vi "stepper driver -- IMS.vi"(6 "Instrument Address":refnum<visa-resource-name>="ASRL2::INSTR", 7 "stepper driver action":T1, 10 "speed IN":dbl, 11 "number":dbl format="%#_13g") -> (1 "stepper motor state OUT":T2, 2 "speed":dbl, 3 "number out":dbl)   [LabVIEW 2018]
uses:
  stepper motor state.ctl
  stepper driver action.ctl
  internal stepper driver state -- IMS.ctl
  Q - not nan -- integer.vi
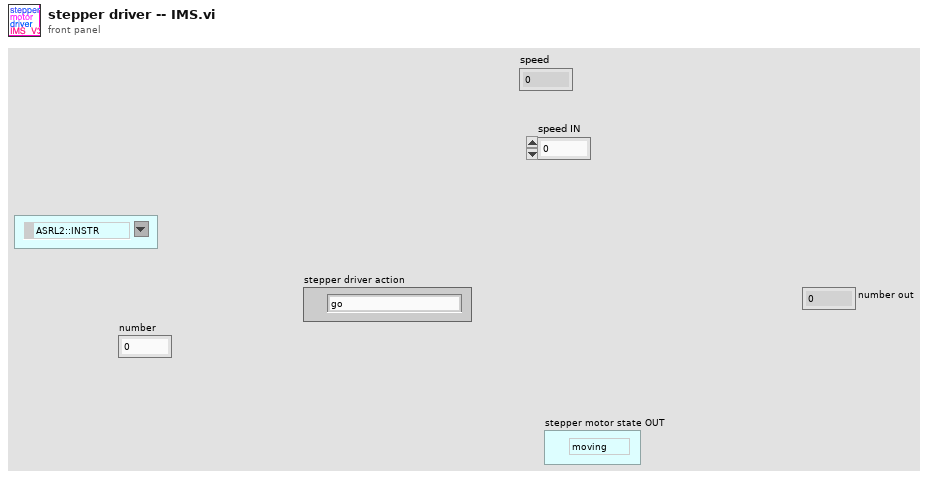
[diagram p1: front panel]
types:
  T1 = typedef "stepper driver action.ctl" = enum16{"go", "void", "stop", "check", "init", "sync", "set", "set speed", "--check status", "--check value"}
  T2 = typedef "stepper motor state.ctl" = enum16{"moving", "stopped"}
  T3 = typedef "internal stepper driver state -- IMS.ctl" = cluster{"VISA address":refnum<visa-resource-name>, "stepper motor state":T2, "Motor Address":u32, "speed":i32, "target position":dbl, "current position":dbl}
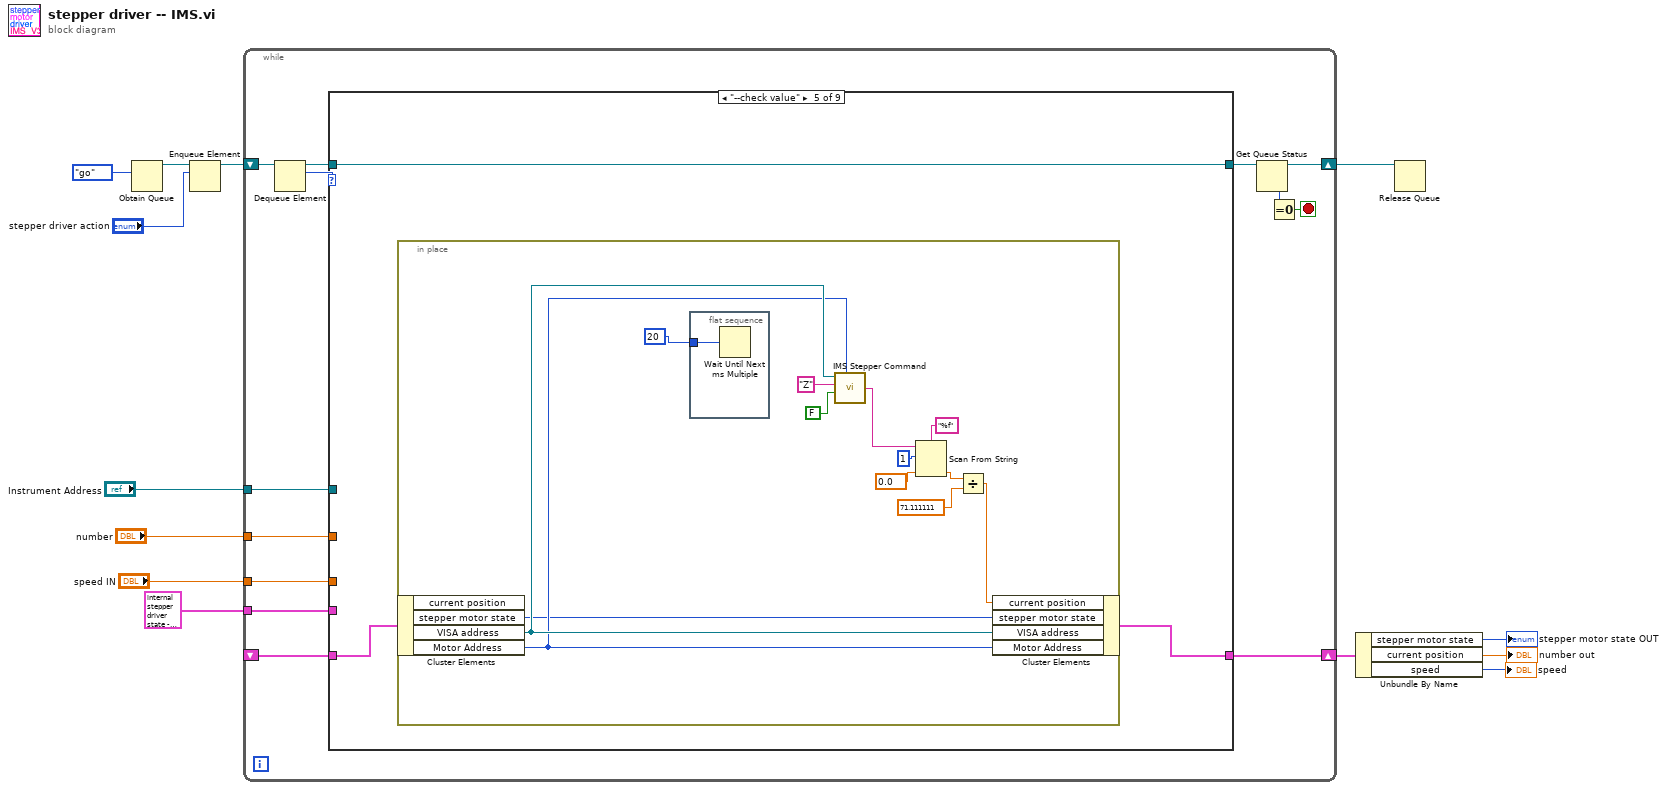
[diagram p0: block diagram]
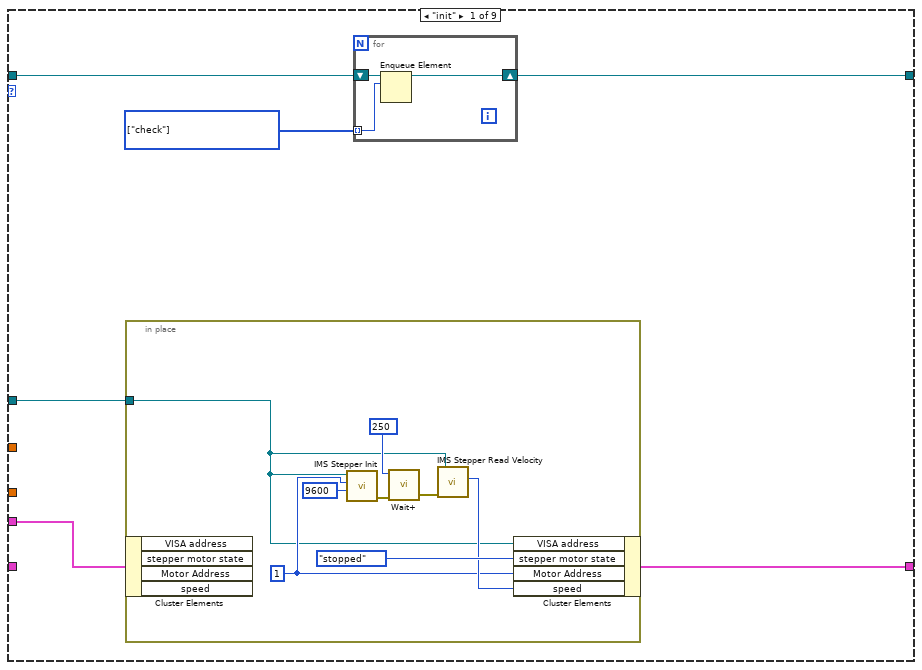
[diagram p2: hidden frame]
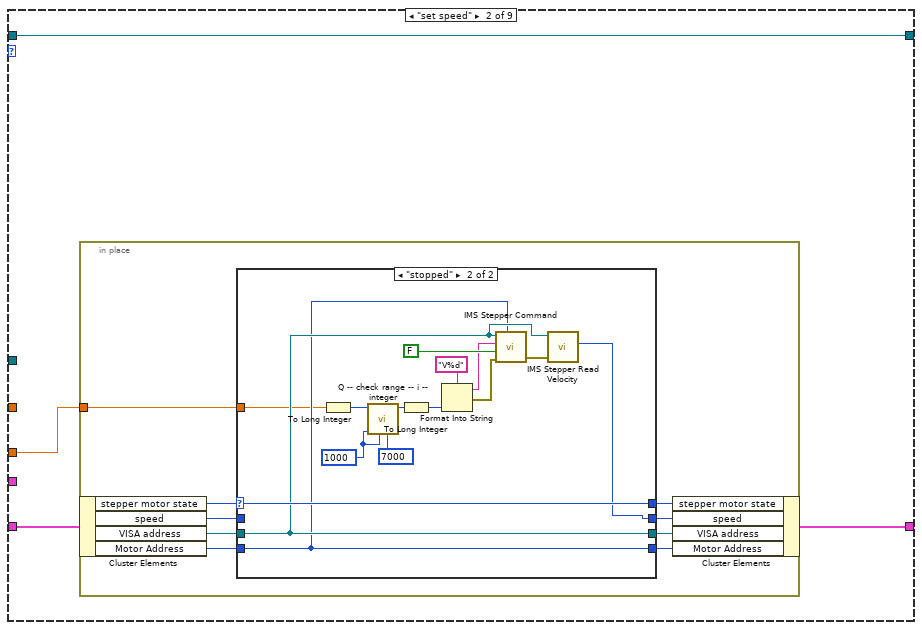
[diagram p3: hidden frame]
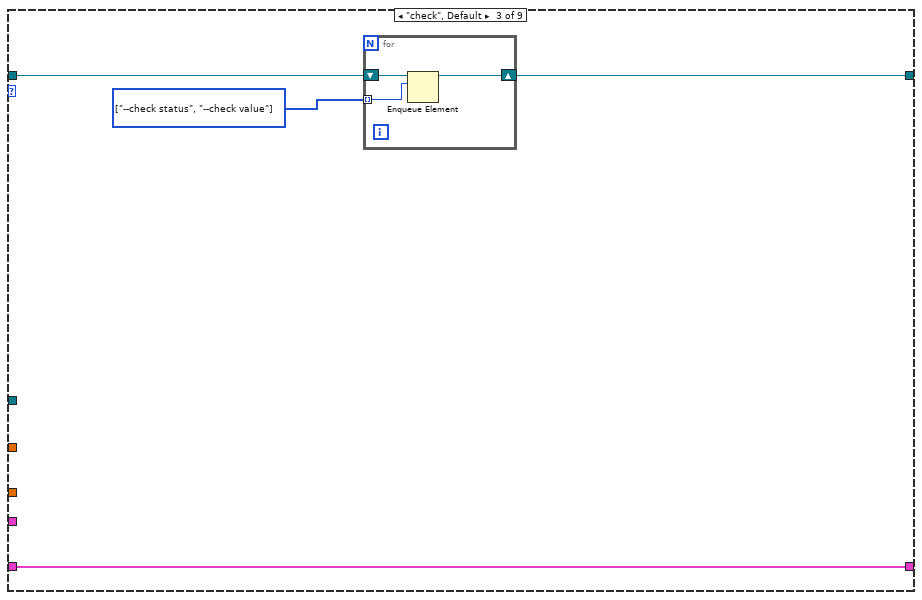
[diagram p5: hidden frame]
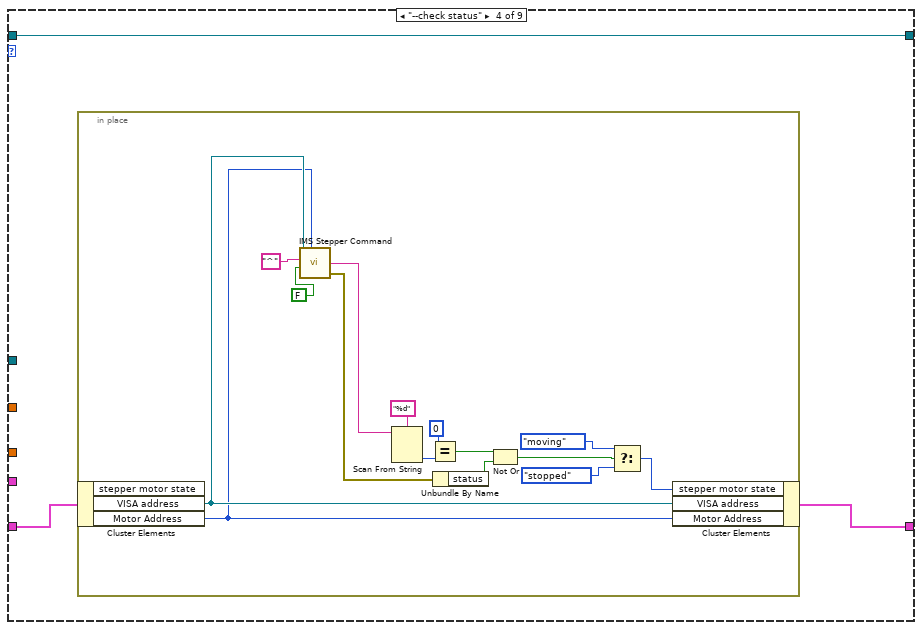
[diagram p6: hidden frame]
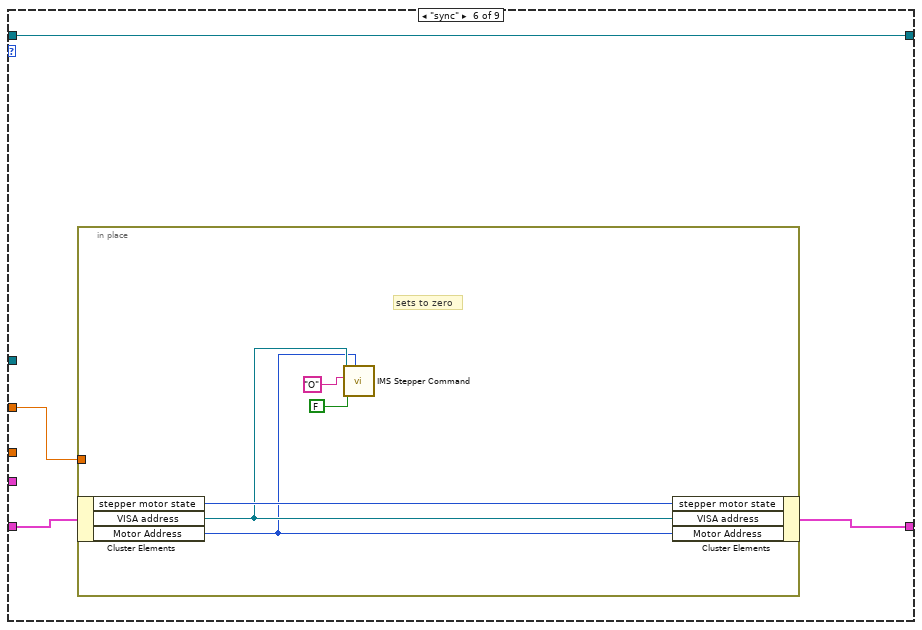
[diagram p7: hidden frame]
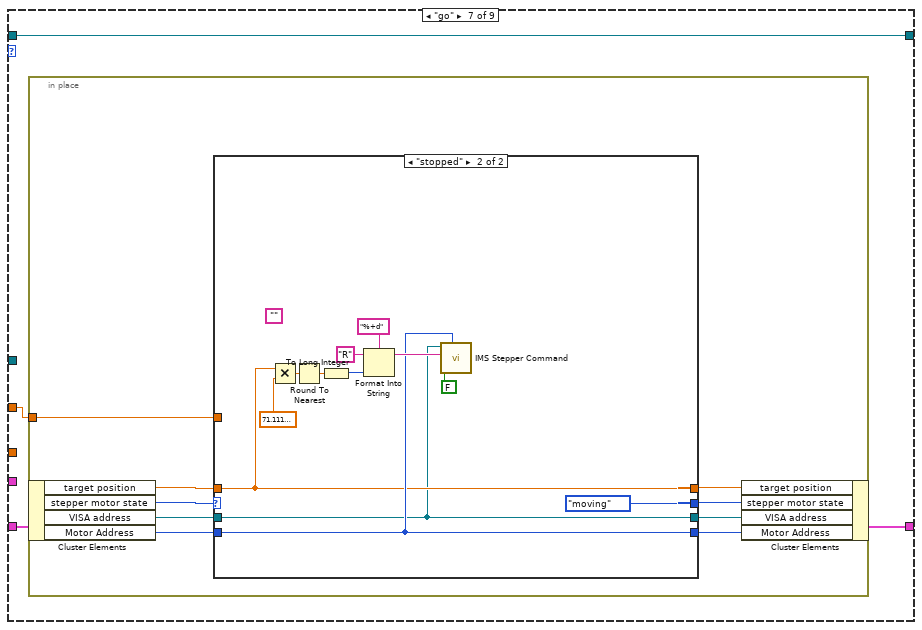
[diagram p8: hidden frame]
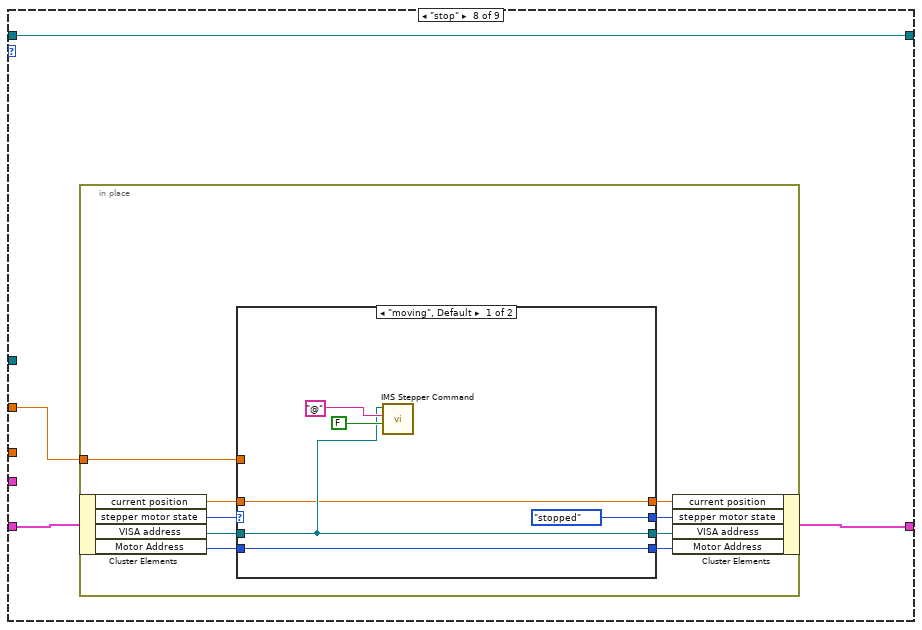
[diagram p10: hidden frame]
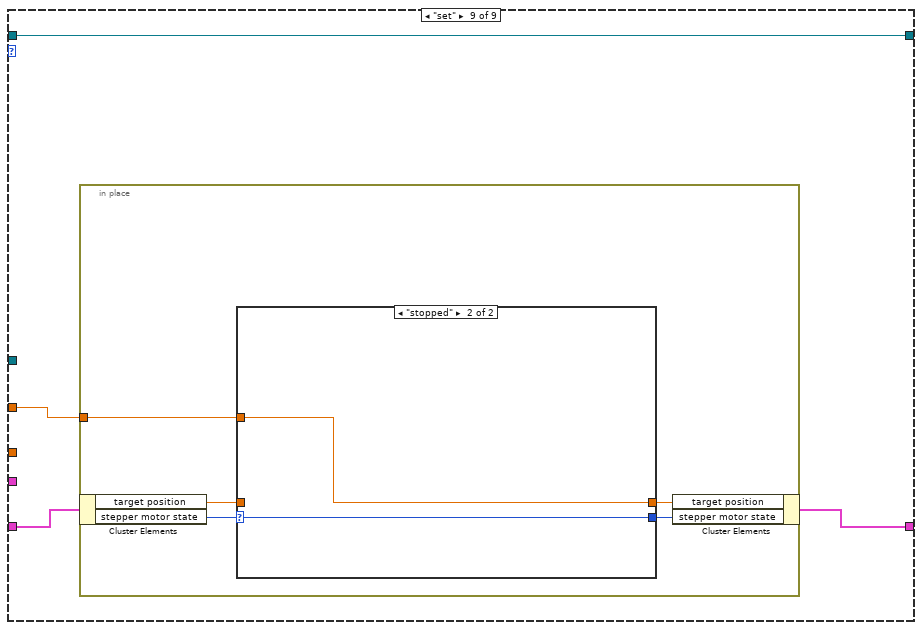
[diagram p12: hidden frame]
diagram:
  n1 = Obtain Queue(element data type=stepper_driver_action."go" ("stepper driver action")) -> (queue out=w8:refnum<queue>)  [unwired: 4 in, 2 out]
  n2 = Enqueue Element(queue=w8, element="stepper driver action") -> (queue out=w7:refnum<queue>)  [unwired: 2 in, 2 out]
  n3 = while {
    shift-right: [w26] -> w10
    shift-left: _ -> [w25]
    shift-right: [w18] -> w6
    shift-left: w7 -> [w22]
    tunnel: T3 {"VISA address"="GPIB0::25::INSTR", "stepper motor state"=enum."stopped", "Motor Address"=0, "speed"=0, "target position"=0.0, "current position"=0.0} ("internal stepper driver state IMS") -> [w24]
    tunnel: "number" -> [w23]
    tunnel: "Instrument Address" -> [w15]
    tunnel: "speed IN" -> [w14]
    stop <- w16 stop-if-true
    n4 = Dequeue Element(queue=w22) -> (queue out=w21:refnum<queue>, element=w20:T1)  [unwired: 2 in, 2 out]
    n5 = case shown="\"--check value\"" w20 {
      tunnel: [w31 w45 w79 w84 w102 w119 w128 w157 w180] -> w26
      tunnel: w25 -> [_ w46 w79 w85 w103 w120 w129 w158 w181]
      tunnel: [w29 w47 w77 w83 w101 w121 w130 w159 w182] -> w19
      tunnel: w21 -> [w30 w47 w78 w83 w101 w121 w130 w159 w182]
      tunnel: w24 -> [w32 _ _ _ _ _ _ _ _]
      tunnel: w23 -> [_ _ _ _ _ w118 w127 w156 w179]
      tunnel: w15 -> [w27 _ _ _ _ _ _ _ _]
      tunnel: w14 -> [_ w44 _ _ _ _ _ _ _]
      frame "init" {
        w28 = T1[] [enum."check"] items=["go", "void", "stop", "check", "init", "sync", "set", "set speed", "--check status", "--check value"] ("action list IN")
        n6 = in-place {
          in-place-border: w27 -> [w36]
          w37 = u32 1 ("Motor Address")
          n7 = in-place-cluster #1(w32) -> ()  [unwired: 4 out]
          n8 = call "IMS Stepper Init.vi"("Baud Rate"=u32 9600, "Motor Number"=w37, "Instrument Address"=w36) -> ("error out"=w42:errorcluster)  [unwired: 1 in, 1 out]
          n9 = call "Wait+.vi"("Error In"=w42, "milliseconds to wait"=u32 250) -> ("Error Out"=w41:errorcluster)  [unwired: 4 in, 1 out]
          n10 = call "IMS Stepper Read Velocity.vi"("error in (no error)"=w41, "Instrument Address"=w36) -> ("Velocity"=w38:i32)  [unwired: 3 in, 2 out]
          n11 = in-place-cluster #1("VISA address"=w36, "stepper motor state"=stepper_motor_state."stopped", "Motor Address"=w37, "speed"=w38) -> (w31:T3)
        }
        n12 = for {
          shift-right: [w34] -> w29
          shift-left: w30 -> [w35]
          tunnel: w28 -> [w33] mode=indexing
          n13 = Enqueue Element(queue=w35, element=w33) -> (queue out=w34:refnum<queue>)  [unwired: 2 in, 2 out]
        }
      }
      frame "set speed" {
        n14 = in-place {
          in-place-border: w44 -> [w56]
          n15 = in-place-cluster #2(w46) -> ("stepper motor state"=w52:T2, "speed"=w51:i32, "VISA address"=w54:refnum<visa-resource-name>, "Motor Address"=w53:u32)
          n16 = case shown="\"stopped\"" w52 {
            selector: w52 -> [w57 w73]
            tunnel: w56 -> [_ w62]
            tunnel: [w60 w64] -> w55
            tunnel: w54 -> [w59 w65]
            tunnel: w53 -> [w58 w63]
            tunnel: w51 -> [w60 _]
            tunnel: [w59 w65] -> w50
            tunnel: [w58 w63] -> w49
            tunnel: [w57 w73] -> w48
            frame "moving", Default {
            }
            frame "stopped" {
              w75 = 1000 ("lower limit")
              n17 = To Long Integer(number=w62) -> (32bit integer=w61:i32)
              n18 = call "Q -- check range -- i -- integer.vi"("upper"=7000 ("x"), "lower"=w75, "default"=w75, "number"=w61) -> ("number in range"=w67:i32)  [unwired: 5 in, 2 out]
              n19 = To Long Integer(number=w67) -> (32bit integer=w66:i32)
              n20 = Format Into String(format string="V%d", w66) -> (resulting string=w70:string, error out=w69:errorcluster)  [unwired: 2 in]
              n21 = call "IMS Stepper Command.vi"("Instrument Address"=w65, "Motor Number"=w63, "Command"=w70, "Mode"=FALSE, "error in (no error)"=w69) -> ("error out"=w68:errorcluster)  [unwired: 1 in, 2 out]
              n22 = call "IMS Stepper Read Velocity.vi"("error in (no error)"=w68, "Instrument Address"=w65) -> ("Velocity"=w64:i32)  [unwired: 3 in, 2 out]
            }
          }
          n23 = in-place-cluster #2("stepper motor state"=w48, "speed"=w55, "VISA address"=w50, "Motor Address"=w49) -> (w45:T3)
        }
      }
      frame "check", Default {
        w76 = T1[] [enum."--check status", enum."--check value"] items=["go", "void", "stop", "check", "init", "sync", "set", "set speed", "--check status", "--check value"] ("action list IN")
        n24 = for {
          shift-right: [w81] -> w77
          shift-left: w78 -> [w82]
          tunnel: w76 -> [w80] mode=indexing
          n25 = Enqueue Element(queue=w82, element=w80) -> (queue out=w81:refnum<queue>)  [unwired: 2 in, 2 out]
        }
      }
      frame "--check status" {
        n26 = in-place {
          n27 = in-place-cluster #3(w85) -> ("VISA address"=w88:refnum<visa-resource-name>, "Motor Address"=w87:u32)  [unwired: 1 out]
          n28 = call "IMS Stepper Command.vi"("Instrument Address"=w88, "Motor Number"=w87, "Command"="^", "Mode"=FALSE) -> ("Response"=w95:string, "error out"=w86:errorcluster)  [unwired: 2 in, 1 out]
          n29 = Scan From String(format string="%d", input string=w95) -> (output 1=w96:i32)  [unwired: 3 in, 3 out]
          n30 = Equal?(x=0, y=w96) -> (x = y?=w97:bool)
          n31 = Unbundle By Name(w86) -> ("status"=w98:bool)
          n32 = Not Or(1:w98, 2:w97) -> (0:w90:bool)
          n33 = Select(t=stepper_motor_state."moving" ("stepper motor state"), s=w90, f=stepper_motor_state."stopped" ("stepper motor state")) -> (s? t:f=w89:T2)
          n34 = in-place-cluster #3("stepper motor state"=w89, "VISA address"=w88, "Motor Address"=w87) -> (w84:T3)
        }
      }
      frame "--check value" {
        n35 = in-place {
          n36 = in-place-cluster #4(w103) -> ("stepper motor state"=w104:T2, "VISA address"=w108:refnum<visa-resource-name>, "Motor Address"=w107:u32)  [unwired: 1 out]
          n37 = flat-sequence {
            tunnel: u32 20 ("millisecond multiple") -> [w117]
            frame #0 {
              n38 = Wait Until Next ms Multiple(millisecond multiple=w117) -> ()  [unwired: 1 out]
            }
          }
          n39 = call "IMS Stepper Command.vi"("Instrument Address"=w108, "Motor Number"=w107, "Command"="Z", "Mode"=FALSE) -> ("Response"=w113:string)  [unwired: 2 in, 2 out]
          n40 = Scan From String(format string="%f", input string=w113, initial scan location=u32 1, default 1=0.0 ("default value 1")) -> (output 1=w115:dbl)  [unwired: 1 in, 3 out]
          n41 = Divide(x=w115, y=71.111111) -> (x/y=w106:dbl)
          n42 = in-place-cluster #4("current position"=w106, "stepper motor state"=w104, "VISA address"=w108, "Motor Address"=w107) -> (w102:T3)
        }
      }
      frame "sync" {
        n43 = in-place {
          in-place-border: w118 -> [_]
          # "sets to zero"
          n44 = in-place-cluster #5(w120) -> ("stepper motor state"=w126:T2, "VISA address"=w123:refnum<visa-resource-name>, "Motor Address"=w122:u32)
          n45 = call "IMS Stepper Command.vi"("Instrument Address"=w123, "Motor Number"=w122, "Command"="O", "Mode"=FALSE) -> ()  [unwired: 2 in, 3 out]
          n46 = in-place-cluster #5("stepper motor state"=w126, "VISA address"=w123, "Motor Address"=w122) -> (w119:T3)
        }
      }
      frame "go" {
        n47 = in-place {
          in-place-border: w127 -> [w139]
          n48 = in-place-cluster #6(w129) -> ("target position"=w133:dbl, "stepper motor state"=w136:T2, "VISA address"=w138:refnum<visa-resource-name>, "Motor Address"=w137:u32)
          n49 = case shown="\"stopped\"" w136 {
            selector: w136 -> [w140 _]
            tunnel: w139 -> [_ _]
            tunnel: w138 -> [w143 w145]
            tunnel: w137 -> [w142 w147]
            tunnel: [w143 w145] -> w135
            tunnel: [w142 w147] -> w134
            tunnel: w133 -> [w141 w146]
            tunnel: [w140 stepper_motor_state."moving" ("stepper motor state")] -> w132
            tunnel: [w141 w146] -> w131
            frame "moving", Default {
            }
            frame "stopped" {
              (unwired) ""
              n50 = Multiply(x=w146, y=71.11111111) -> (x*y=w153:dbl)
              n51 = Round To Nearest(number=w153) -> (nearest integer value=w151:dbl)
              n52 = To Long Integer(number=w151) -> (32bit integer=w152:i32)
              n53 = Format Into String(format string="%+d", initial string="R", w152) -> (resulting string=w148:string)  [unwired: 1 in, 1 out]
              n54 = call "IMS Stepper Command.vi"("Instrument Address"=w145, "Motor Number"=w147, "Command"=w148, "Mode"=FALSE) -> ()  [unwired: 2 in, 3 out]
            }
          }
          n55 = in-place-cluster #6("target position"=w131, "stepper motor state"=w132, "VISA address"=w135, "Motor Address"=w134) -> (w128:T3)
        }
      }
      frame "stop" {
        n56 = in-place {
          in-place-border: w156 -> [w168]
          n57 = in-place-cluster #7(w158) -> ("current position"=w160:dbl, "stepper motor state"=w165:T2, "VISA address"=w167:refnum<visa-resource-name>, "Motor Address"=w166:u32)
          n58 = case shown="\"moving\", Default" w165 {
            selector: w165 -> [_ w176]
            tunnel: w168 -> [_ _]
            tunnel: w167 -> [w170 w178]
            tunnel: w166 -> [w174 w177]
            tunnel: [w170 w178] -> w164
            tunnel: [w174 w177] -> w163
            tunnel: [stepper_motor_state."stopped" ("stepper motor state") w176] -> w162
            tunnel: [w169 w175] -> w161
            tunnel: w160 -> [w169 w175]
            frame "moving", Default {
              n59 = call "IMS Stepper Command.vi"("Instrument Address"=w170, "Command"="@", "Mode"=FALSE) -> ()  [unwired: 3 in, 3 out]
            }
            frame "stopped" {
            }
          }
          n60 = in-place-cluster #7("current position"=w161, "stepper motor state"=w162, "VISA address"=w164, "Motor Address"=w163) -> (w157:T3)
        }
      }
      frame "set" {
        n61 = in-place {
          in-place-border: w179 -> [w187]
          n62 = in-place-cluster #8(w181) -> ("target position"=w183:dbl, "stepper motor state"=w186:T2)
          n63 = case shown="\"stopped\"" w186 {
            selector: w186 -> [w189 w191]
            tunnel: w187 -> [_ w190]
            tunnel: [w189 w191] -> w185
            tunnel: [w188 w190] -> w184
            tunnel: w183 -> [w188 _]
            frame "moving", Default {
            }
            frame "stopped" {
            }
          }
          n64 = in-place-cluster #8("target position"=w184, "stepper motor state"=w185) -> (w180:T3)
        }
      }
    }
    n65 = Get Queue Status(queue=w19) -> (queue out=w18:refnum<queue>, # elements in queue=w17:i32)  [unwired: 2 in, 6 out]
    n66 = Equal To 0?(x=w17) -> (x = 0?=w16:bool)
  }
  n67 = Unbundle By Name(w10) -> ("stepper motor state"=→"stepper motor state OUT":T2, "current position"=→"number out":dbl, "speed"=→"speed":i32)
  n68 = Release Queue(queue=w6) -> ()  [unwired: 2 in, 3 out]
